vi "Main.vi"() -> ()   [LabVIEW 2018] (continued)
                n2266 = Insert Into Array(array=string[] [] ("数组"), index=0 ("索引"), new element #1=w3062, new element #2=w3061, new element #3=w3060) -> (w3066:string[])
                n2267 = Bundle By Name(cluster=cluster{"Data":string[], "State":T1} {"Data"=[], "State"=enum."PLC通讯初始化"} ("元素"), "Data"=w3066, "State"=状态2."扫码回复") -> (w3067:cluster{"Data":string[], "State":T1})
                n2268 = Enqueue Element(queue=w3056, element=w3067) -> ()  [unwired: 2 in, 3 out]
              }
            }
            n2269 = Unbundle By Name(w2986) -> ("source"=w2985:string)
            n2270 = Concatenate Strings("80扫码异常 ", w2985) -> (w2983:string)
            "ST80扫码请求(事件)" <- FALSE ("ST80扫码请求(事件)")
          }
          event "查询": Value Change {
            n2271 = event-data() -> ()  [unwired: 1 in, 2 out]
            n2272 = flat-sequence {
              tunnel: w3083 -> [w3108]
              tunnel: w3082 -> [w3107]
              tunnel: [w3099] -> w3081
              frame #0 {
                w3084 = cluster{u32, u32}[] [{1985280, 1985280}, {6618880, 6618880}, {1985280, 1985280}, {6618880, 6618880}] ("颜色[4]")
                n2273 = property on="101" class="Bool (严格)"("Colors [4]"=w3084) -> ()  [unwired: 2 in, 2 out]
                n2274 = property on="102" class="Bool (严格)"("Colors [4]"=w3084) -> ()  [unwired: 2 in, 2 out]
                n2275 = property on="202" class="Bool (严格)"("Colors [4]"=w3084) -> ()  [unwired: 2 in, 2 out]
                n2276 = property on="203" class="Bool (严格)"("Colors [4]"=w3084) -> ()  [unwired: 2 in, 2 out]
                n2277 = property on="301" class="Bool (严格)"("Colors [4]"=w3084) -> ()  [unwired: 2 in, 2 out]
                n2278 = property on="302" class="Bool (严格)"("Colors [4]"=w3084) -> ()  [unwired: 2 in, 2 out]
                n2279 = property on="401" class="Bool (严格)"("Colors [4]"=w3084) -> ()  [unwired: 2 in, 2 out]
                n2280 = property on="403" class="Bool (严格)"("Colors [4]"=w3084) -> ()  [unwired: 2 in, 2 out]
                n2281 = property on="502" class="Bool (严格)"("Colors [4]"=w3084) -> ()  [unwired: 2 in, 2 out]
                n2282 = property on="503" class="Bool (严格)"("Colors [4]"=w3084) -> ()  [unwired: 2 in, 2 out]
                n2283 = property on="601" class="Bool (严格)"("Colors [4]"=w3084) -> ()  [unwired: 2 in, 2 out]
                n2284 = property on="602" class="Bool (严格)"("Colors [4]"=w3084) -> ()  [unwired: 2 in, 2 out]
                n2285 = property on="70" class="Bool (严格)"("Colors [4]"=w3084) -> ()  [unwired: 2 in, 2 out]
                n2286 = property on="80" class="Bool (严格)"("Colors [4]"=w3084) -> ()  [unwired: 2 in, 2 out]
              }
              frame #1 {
                n2287 = Concatenate Strings("Where QRCode='" ("查询语句"), "输入需要Rework的一维码：", "'" ("字符串")) -> (w3109:string)
                n2288 = call "SQL_Select.vi"("要读取的列名"=string[] ["Last_Station", "Last_Result"] ("列名"), "表名"="Online", "error in (no error)"=w3107, "查询语句"=w3109, "查询条件"=TRUE, "connection reference"=w3108) -> ("error out"=w3099:errorcluster, "数据"=w3104:string[][])  [unwired: 3 in, 1 out]
                n2289 = Index Array(array=w3104, index (row)=0 ("索引 (行)")) -> (element=w3102:string[])  [unwired: 1 in]
                n2290 = Index Array(array=w3102) -> (element #1=w3101:string, element #2=w3100:string)  [unwired: 2 in]
                n2291 = case shown="\"0\", 默认" w3101 {
                  tunnel: w3100 -> [_ w3117 w3124 w3131 w3138 w3145 w3152 w3159 w3166 w3173 w3180 w3187 w3194 w3201 w3207]
                  tunnel: [w3114 w3116 TRUE w3129 w3136 w3143 w3150 w3157 w3164 w3171 w3178 w3185 w3192 w3199 w3205] -> w3098
                  tunnel: [w3114 w3115 w3123 w3129 w3136 w3143 w3150 w3157 w3164 w3171 w3178 w3185 w3192 w3199 w3205] -> w3097
                  tunnel: [w3114 w3115 w3121 w3130 w3136 w3143 w3150 w3157 w3164 w3171 w3178 w3185 w3192 w3199 w3205] -> w3096
                  tunnel: [w3114 w3115 w3121 w3128 w3137 w3143 w3150 w3157 w3164 w3171 w3178 w3185 w3192 w3199 w3205] -> w3095
                  tunnel: [w3114 w3115 w3121 w3128 w3135 w3144 w3150 w3157 w3164 w3171 w3178 w3185 w3192 w3199 w3205] -> w3094
                  tunnel: [w3114 w3115 w3121 w3128 w3135 w3142 w3151 w3157 w3164 w3171 w3178 w3185 w3192 w3199 w3205] -> w3093
                  tunnel: [w3114 w3115 w3121 w3128 w3135 w3142 w3149 w3158 w3164 w3171 w3178 w3185 w3192 w3199 w3205] -> w3092
                  tunnel: [w3114 w3115 w3121 w3128 w3135 w3142 w3149 w3156 w3165 w3171 w3178 w3185 w3192 w3199 w3205] -> w3091
                  tunnel: [w3114 w3115 w3121 w3128 w3135 w3142 w3149 w3156 w3163 w3172 w3178 w3185 w3192 w3199 w3205] -> w3090
                  tunnel: [w3114 w3115 w3121 w3128 w3135 w3142 w3149 w3156 w3163 w3170 w3179 w3185 w3192 w3199 w3205] -> w3089
                  tunnel: [w3114 w3115 w3121 w3128 w3135 w3142 w3149 w3156 w3163 w3170 w3177 w3186 w3192 w3199 w3205] -> w3088
                  tunnel: [w3114 w3115 w3121 w3128 w3135 w3142 w3149 w3156 w3163 w3170 w3177 w3184 w3193 w3199 w3205] -> w3087
                  tunnel: [w3114 w3115 w3121 w3128 w3135 w3142 w3149 w3156 w3163 w3170 w3177 w3184 w3191 w3200 w3205] -> w3086
                  tunnel: [w3114 w3115 w3121 w3128 w3135 w3142 w3149 w3156 w3163 w3170 w3177 w3184 w3191 FALSE w3206] -> w3085
                  frame "0", Default {
                    w3114 = FALSE
                  }
                  frame "101" {
                    w3115 = FALSE
                    n2292 = case shown="\"OK\", 默认" w3117 {
                      tunnel: [TRUE FALSE] -> w3116
                      frame "OK", Default {
                      }
                      frame "NG" {
                        n2293 = property on="101" class="Bool (严格)"("Colors [4]"=cluster{u32, u32}[] [{16711680, 16711680}, {6618880, 6618880}, {1985280, 1985280}, {6618880, 6618880}] ("颜色[4]")) -> ()  [unwired: 2 in, 2 out]
                      }
                    }
                  }
                  frame "102" {
                    w3121 = FALSE
                    n2294 = case shown="\"NG\"" w3124 {
                      tunnel: [TRUE FALSE] -> w3123
                      frame "OK", Default {
                      }
                      frame "NG" {
                        n2295 = property on="102" class="Bool (严格)"("Colors [4]"=cluster{u32, u32}[] [{16711680, 16711680}, {6618880, 6618880}, {1985280, 1985280}, {6618880, 6618880}] ("颜色[4]")) -> ()  [unwired: 2 in, 2 out]
                      }
                    }
                  }
                  frame "202" {
                    w3129 = TRUE
                    w3128 = FALSE
                    n2296 = case shown="\"NG\"" w3131 {
                      tunnel: [TRUE FALSE] -> w3130
                      frame "OK", Default {
                      }
                      frame "NG" {
                        n2297 = property on="202" class="Bool (严格)"("Colors [4]"=cluster{u32, u32}[] [{16711680, 16711680}, {6618880, 6618880}, {1985280, 1985280}, {6618880, 6618880}] ("颜色[4]")) -> ()  [unwired: 2 in, 2 out]
                      }
                    }
                  }
                  frame "203" {
                    w3136 = TRUE
                    w3135 = FALSE
                    n2298 = case shown="\"NG\"" w3138 {
                      tunnel: [TRUE FALSE] -> w3137
                      frame "OK", Default {
                      }
                      frame "NG" {
                        n2299 = property on="203" class="Bool (严格)"("Colors [4]"=cluster{u32, u32}[] [{16711680, 16711680}, {6618880, 6618880}, {1985280, 1985280}, {6618880, 6618880}] ("颜色[4]")) -> ()  [unwired: 2 in, 2 out]
                      }
                    }
                  }
                  frame "301" {
                    w3143 = TRUE
                    w3142 = FALSE
                    n2300 = case shown="\"NG\"" w3145 {
                      tunnel: [TRUE FALSE] -> w3144
                      frame "OK", Default {
                      }
                      frame "NG" {
                        n2301 = property on="301" class="Bool (严格)"("Colors [4]"=cluster{u32, u32}[] [{16711680, 16711680}, {6618880, 6618880}, {1985280, 1985280}, {6618880, 6618880}] ("颜色[4]")) -> ()  [unwired: 2 in, 2 out]
                      }
                    }
                  }
                  frame "302" {
                    w3150 = TRUE
                    w3149 = FALSE
                    n2302 = case shown="\"NG\"" w3152 {
                      tunnel: [TRUE FALSE] -> w3151
                      frame "OK", Default {
                      }
                      frame "NG" {
                        n2303 = property on="302" class="Bool (严格)"("Colors [4]"=cluster{u32, u32}[] [{16711680, 16711680}, {6618880, 6618880}, {1985280, 1985280}, {6618880, 6618880}] ("颜色[4]")) -> ()  [unwired: 2 in, 2 out]
                      }
                    }
                  }
                  frame "401" {
                    w3157 = TRUE
                    w3156 = FALSE
                    n2304 = case shown="\"NG\"" w3159 {
                      tunnel: [TRUE FALSE] -> w3158
                      frame "OK", Default {
                      }
                      frame "NG" {
                        n2305 = property on="401" class="Bool (严格)"("Colors [4]"=cluster{u32, u32}[] [{16711680, 16711680}, {6618880, 6618880}, {1985280, 1985280}, {6618880, 6618880}] ("颜色[4]")) -> ()  [unwired: 2 in, 2 out]
                      }
                    }
                  }
                  frame "403" {
                    w3163 = FALSE
                    w3164 = TRUE
                    n2306 = case shown="\"NG\"" w3166 {
                      tunnel: [TRUE FALSE] -> w3165
                      frame "OK", Default {
                      }
                      frame "NG" {
                        n2307 = property on="403" class="Bool (严格)"("Colors [4]"=cluster{u32, u32}[] [{16711680, 16711680}, {6618880, 6618880}, {1985280, 1985280}, {6618880, 6618880}] ("颜色[4]")) -> ()  [unwired: 2 in, 2 out]
                      }
                    }
                  }
                  frame "502" {
                    w3170 = FALSE
                    w3171 = TRUE
                    n2308 = case shown="\"NG\"" w3173 {
                      tunnel: [TRUE FALSE] -> w3172
                      frame "OK", Default {
                      }
                      frame "NG" {
                        n2309 = property on="502" class="Bool (严格)"("Colors [4]"=cluster{u32, u32}[] [{16711680, 16711680}, {6618880, 6618880}, {1985280, 1985280}, {6618880, 6618880}] ("颜色[4]")) -> ()  [unwired: 2 in, 2 out]
                      }
                    }
                  }
                  frame "503" {
                    w3177 = FALSE
                    w3178 = TRUE
                    n2310 = case shown="\"NG\"" w3180 {
                      tunnel: [TRUE FALSE] -> w3179
                      frame "OK", Default {
                      }
                      frame "NG" {
                        n2311 = property on="503" class="Bool (严格)"("Colors [4]"=cluster{u32, u32}[] [{16711680, 16711680}, {6618880, 6618880}, {1985280, 1985280}, {6618880, 6618880}] ("颜色[4]")) -> ()  [unwired: 2 in, 2 out]
                      }
                    }
                  }
                  frame "601" {
                    w3184 = FALSE
                    w3185 = TRUE
                    n2312 = case shown="\"NG\"" w3187 {
                      tunnel: [TRUE FALSE] -> w3186
                      frame "OK", Default {
                      }
                      frame "NG" {
                        n2313 = property on="601" class="Bool (严格)"("Colors [4]"=cluster{u32, u32}[] [{16711680, 16711680}, {6618880, 6618880}, {1985280, 1985280}, {6618880, 6618880}] ("颜色[4]")) -> ()  [unwired: 2 in, 2 out]
                      }
                    }
                  }
                  frame "602" {
                    w3191 = FALSE
                    w3192 = TRUE
                    n2314 = case shown="\"NG\"" w3194 {
                      tunnel: [TRUE FALSE] -> w3193
                      frame "OK", Default {
                      }
                      frame "NG" {
                        n2315 = property on="602" class="Bool (严格)"("Colors [4]"=cluster{u32, u32}[] [{16711680, 16711680}, {6618880, 6618880}, {1985280, 1985280}, {6618880, 6618880}] ("颜色[4]")) -> ()  [unwired: 2 in, 2 out]
                      }
                    }
                  }
                  frame "70" {
                    w3199 = TRUE
                    n2316 = case shown="\"NG\"" w3201 {
                      tunnel: [TRUE FALSE] -> w3200
                      frame "OK", Default {
                      }
                      frame "NG" {
                        n2317 = property on="70" class="Bool (严格)"("Colors [4]"=cluster{u32, u32}[] [{16711680, 16711680}, {6618880, 6618880}, {1985280, 1985280}, {6618880, 6618880}] ("颜色[4]")) -> ()  [unwired: 2 in, 2 out]
                      }
                    }
                  }
                  frame "80" {
                    w3205 = TRUE
                    n2318 = case shown="\"NG\"" w3207 {
                      tunnel: [TRUE FALSE] -> w3206
                      frame "OK", Default {
                      }
                      frame "NG" {
                        n2319 = property on="80" class="Bool (严格)"("Colors [4]"=cluster{u32, u32}[] [{16711680, 16711680}, {6618880, 6618880}, {1985280, 1985280}, {6618880, 6618880}] ("颜色[4]")) -> ()  [unwired: 2 in, 2 out]
                      }
                    }
                  }
                }
                n2320 = local write "101"(w3098) -> ()
                n2321 = local write "102"(w3097) -> ()
                n2322 = local write "202"(w3096) -> ()
                n2323 = local write "203"(w3095) -> ()
                n2324 = local write "301"(w3094) -> ()
                n2325 = local write "302"(w3093) -> ()
                n2326 = local write "401"(w3092) -> ()
                n2327 = local write "403"(w3091) -> ()
                n2328 = local write "502"(w3090) -> ()
                n2329 = local write "503"(w3089) -> ()
                n2330 = local write "601"(w3088) -> ()
                n2331 = local write "602"(w3087) -> ()
                n2332 = local write "70"(w3086) -> ()
                n2333 = local write "80"(w3085) -> ()
              }
            }
          }
          event "确定Rework": Value Change {
            n2334 = event-data() -> ()  [unwired: 1 in, 2 out]
            n2335 = stacked-sequence {
              seq-local: [w3215 _] -> [_ w3241]
              tunnel: w3214 -> [w3225 w3246]
              tunnel: w3213 -> [w3224 w3245]
              tunnel: [_ w3244] -> w3212
              frame #0 {
                n2336 = local read "输入需要Rework的一维码："() -> (w3220:string)
                n2337 = Concatenate Strings("Where QRCode='" ("查询语句"), w3220, "'" ("字符串")) -> (w3219:string)
                n2338 = call "SQL_Select.vi"("表名"="Online", "error in (no error)"=w3224, "查询语句"=w3219, "查询条件"=TRUE, "connection reference"=w3225) -> ("数据"=w3218:string[][])  [unwired: 4 in, 2 out]
                n2339 = Matrix Size(0:w3218) -> (1:w3217:i32)  [unwired: 1 out]
                n2340 = Equal?(x=w3217, y=0) -> (x = y?=w3215:bool)
              }
              frame #1 {
                n2341 = Insert Into Array(array=bool[] [] ("数组"), index=0 ("索引"), new element #1="70", new element #2="602", new element #3="601", new element #4="503", new element #5="502", new element #6="403", new element #7="401", new element #8="302", new element #9="301", new element #10="203", new element #11="202", new element #12="102", new element #13="101", new element #14="80") -> (w3250:bool[])
                n2342 = Search 1D Array(1D array=w3250, element=TRUE ("元素")) -> (index of element=w3247:i32)  [unwired: 1 in]
                n2343 = Equal?(x=w3247, y=-1) -> (x = y?=w3243:bool)
                n2344 = Or(x=w3243, y=w3241) -> (x .or. y?=w3242:bool)
                n2345 = case shown="假" w3242 {
                  tunnel: w3247 -> [w3290 _]
                  tunnel: w3246 -> [w3289 _]
                  tunnel: w3245 -> [w3288 w3392]
                  tunnel: [w3258 w3392] -> w3244
                  frame False {
                    w3263 = "Rework_List" ("表名")
                    w3261 = 0 ("索引 (行)")
                    w3273 = "Online" ("表名")
                    n2346 = case shown="13" w3290 {
                      tunnel: w3289 -> [w3351 w3353 w3357 w3360 w3363 w3366 w3369 w3372 w3375 w3378 w3381 w3384 w3386 w3389]
                      tunnel: w3288 -> [w3350 w3352 w3356 w3359 w3362 w3365 w3368 w3371 w3374 w3377 w3380 w3383 w3385 w3388]
                      tunnel: [w3350 w3352 w3356 w3359 w3362 w3365 w3368 w3371 w3374 w3377 w3380 w3383 w3385 w3388] -> w3276
                      tunnel: [w3351 w3353 w3357 w3360 w3363 w3366 w3369 w3372 w3375 w3378 w3381 w3384 w3386 w3389] -> w3277
                      tunnel: ["70" "602" "601" "503" "502" "403" "401" "302" "301" "203" "202" "102" "101" "80"] -> w3253
                      frame 0, Default {
                      }
                      frame 1 {
                      }
                      frame 2 {
                      }
                      frame 3 {
                      }
                      frame 4 {
                      }
                      frame 5 {
                      }
                      frame 6 {
                      }
                      frame 7 {
                      }
                      frame 8 {
                      }
                      frame 9 {
                      }
                      frame 10 {
                      }
                      frame 11 {
                      }
                      frame 12 {
                      }
                      frame 13 {
                      }
                    }
                    n2347 = local read "输入需要Rework的一维码："() -> (w3259:string)
                    n2348 = Concatenate Strings("Where QRCode='" ("查询语句"), w3259, "'" ("字符串")) -> (w3260:string)
                    n2349 = call "SQL_Select.vi"("要读取的列名"=string[] ["Last_Station"], "表名"=w3273, "error in (no error)"=w3276, "查询语句"=w3260, "查询条件"=TRUE, "connection reference"=w3277) -> ("error out"=w3274:errorcluster, "数据"=w3272:string[][], "connection reference out"=w3275:T12)  [unwired: 3 in]
                    n2350 = Index Array(array=w3272, index (row)=w3261, index (col)=w3261) -> (element=w3254:string)
                    n2351 = Insert Into Array(array=string[] [] ("数组"), index=0 ("索引"), new element #1=w3253, new element #2="OK" ("新元素/子数组"), new element #3="T" ("新元素/子数组")) -> (w3286:string[])
                    n2352 = call "SQL_Update.vi"("查询语句"=w3260, "表名"=w3273, "error in (no error)"=w3274, "列名对应的值"=w3286, "列名"=string[] ["Last_Station", "Last_Result", "Rework_Status"], "connection reference"=w3275) -> ("error out"=w3271:errorcluster, "connection reference 2"=w3270:T12)  [unwired: 4 in]
                    n2353 = call "SQL_Select.vi"("表名"=w3263, "error in (no error)"=w3271, "查询语句"=w3260, "查询条件"=TRUE, "connection reference"=w3270) -> ("error out"=w3264:errorcluster, "数据"=w3268:string[][], "connection reference out"=w3265:T12)  [unwired: 4 in]
                    n2354 = call "Rework_Calculate-1.vi"("Rework站号"=w3253, "当前站号"=w3254) -> ("Data"=w3255:string[], "Rework_List"=w3256:string[], "跨站"=w3257:bool)  [unwired: 7 in]
                    n2355 = Matrix Size(0:w3268) -> (1:w3267:i32)  [unwired: 1 out]
                    n2356 = Equal To 0?(x=w3267) -> (x = 0?=w3266:bool)
                    n2357 = case shown="假" w3257 {
                      tunnel: w3266 -> [w3309 _]
                      tunnel: w3265 -> [w3308 w3345]
                      tunnel: w3264 -> [w3307 w3346]
                      tunnel: w3255 -> [w3306 _]
                      tunnel: w3256 -> [w3305 _]
                      tunnel: w3263 -> [w3304 _]
                      tunnel: w3260 -> [w3300 _]
                      tunnel: w3259 -> [w3293 _]
                      tunnel: [w3292 w3346] -> w3258
                      tunnel: [w3291 w3345] -> _
                      frame False {
                        w3294 = "Rework" ("表名")
                        n2358 = case shown="真" w3309 {
                          tunnel: w3308 -> [w3331 w3344]
                          tunnel: w3307 -> [w3330 w3343]
                          tunnel: w3306 -> [w3328 w3338]
                          tunnel: w3305 -> [w3329 w3341]
                          tunnel: w3304 -> [w3327 w3342]
                          tunnel: w3293 -> [_ w3336]
                          tunnel: [w3325 w3333] -> w3302
                          tunnel: [w3324 w3332] -> w3301
                          tunnel: w3300 -> [w3326 _]
                          frame False {
                            n2359 = call "SQL_Update.vi"("查询语句"=w3326, "表名"=w3327, "error in (no error)"=w3330, "列名对应的值"=w3328, "列名"=w3329, "connection reference"=w3331) -> ("error out"=w3324:errorcluster, "connection reference 2"=w3325:T12)  [unwired: 4 in]
                          }
                          frame True {
                            n2360 = Insert Into Array(array=w3341, index=0 ("索引"), new element="QRCode" ("新元素/子数组")) -> (w3335:string[])
                            n2361 = Insert Into Array(array=w3338, index=0 ("索引"), new element=w3336) -> (w3334:string[])
                            n2362 = call "SQL_Insert.vi"("表名"=w3342, "error in (no error)"=w3343, "值"=w3334, "列名"=w3335, "connection reference"=w3344) -> ("error out"=w3332:errorcluster, "connection reference 2"=w3333:T12)  [unwired: 5 in]
                          }
                        }
                        n2363 = call "SQL_Select.vi"("表名"=w3294, "error in (no error)"=w3301, "查询语句"=w3300, "查询条件"=TRUE, "connection reference"=w3302) -> ("error out"=w3295:errorcluster, "数据"=w3299:string[][], "connection reference out"=w3296:T12)  [unwired: 4 in]
                        n2364 = Matrix Size(0:w3299) -> (1:w3298:i32)  [unwired: 1 out]
                        n2365 = Equal To 0?(x=w3298) -> (x = 0?=w3297:bool)
                        n2366 = case shown="真" w3297 {
                          tunnel: w3296 -> [w3310 w3323]
                          tunnel: w3295 -> [w3311 w3322]
                          tunnel: w3294 -> [_ w3321]
                          tunnel: w3293 -> [_ w3319]
                          tunnel: [w3311 w3315] -> w3292
                          tunnel: [w3310 w3312] -> w3291
                          frame False {
                          }
                          frame True {
                            n2367 = Format Date/Time String(time format string (%c)="%Y-%m-%d_%H:%M" ("时间格式字符串(%c)")) -> (date/time string=w3313:string)  [unwired: 2 in]
                            n2368 = Insert Into Array(array=string[] [] ("数组"), index=0 ("索引"), new element #1=w3319, new element #2=w3313) -> (w3316:string[])
                            n2369 = call "SQL_Insert.vi"("表名"=w3321, "error in (no error)"=w3322, "值"=w3316, "列名"=string[] ["QRCode", "Online_Time"], "connection reference"=w3323) -> ("error out"=w3315:errorcluster, "connection reference 2"=w3312:T12)  [unwired: 5 in]
                          }
                        }
                      }
                      frame True {
                      }
                    }
                    n2370 = case shown="错误" w3258 {
                      tunnel: ["Rework成功！" ("Rework状态") "Rework失败！" ("Rework状态")] -> w3262
                      frame No Error {
                      }
                      frame Error {
                      }
                    }
                    "Rework状态" <- w3262
                  }
                  frame True {
                    n2371 = local write "Rework状态"("该条码不存在！" ("Rework状态")) -> ()
                  }
                }
              }
            }
          }
        }
        n2372 = event shown="[2] \"ST70数据读取(事件)\": 值改变" {
          selector: _ -> [_ _ _]
          dyn-events: _ -> [_ _ _]
          timeout: 10 -> [_ _ _]
          tunnel: w763 -> [_ w788 w836]
          tunnel: w762 -> [_ w787 w835]
          tunnel: w761 -> [_ w786 w837]
          tunnel: w760 -> [_ _ w838]
          event Timeout {
            n2373 = event-data() -> ()  [unwired: 1 in, 3 out]
          }
          event "ST70扫码请求(事件)": Value Change {
            n2374 = event-data() -> ()  [unwired: 1 in, 1 out]
            n2375 = local read "70二维码"() -> (w815:string)
            n2376 = Concatenate Strings("Where QRCode='" ("查询语句"), w815, "'" ("字符串")) -> (w803:string)
            n2377 = call "SQL_Select.vi"("要读取的列名"=string[] ["Last_Station", "Last_Result"], "表名"="Online", "error in (no error)"=w787, "查询语句"=w803, "查询条件"=TRUE, "connection reference"=w788) -> ("error out"=w784:errorcluster, "数据"=w804:string[][])  [unwired: 3 in, 1 out]
            n2378 = case shown="无错误" w784 {
              tunnel: w804 -> [w831 _]
              tunnel: ["1" ("右扫码请求回复") "2" ("右扫码请求回复")] -> w807
              tunnel: [w826 w832] -> w808
              tunnel: [w825 w832] -> w809
              frame No Error {
                n2379 = Index Array(array=w831, index (row)=0 ("索引 (行)")) -> (element=w828:string[])  [unwired: 1 in]
                n2380 = Index Array(array=w828, index #1=0 ("索引 (行)")) -> (element #1=w826:string, element #2=w825:string)  [unwired: 1 in]
                "上一站号 (70)" <- w826
                "上一站结果 (70)" <- w825
              }
              frame Error {
                w832 = ""
              }
            }
            n2381 = Insert Into Array(array=string[] [] ("数组"), index=0 ("索引"), new element #1=w807, new element #2=w808, new element #3=w809) -> (w806:string[])
            n2382 = Format Date/Time String(time format string (%c)="%Y-%m-%d" ("时间格式字符串(%c)")) -> (date/time string=w810:string)  [unwired: 2 in]
            n2383 = Get Date/Time String() -> (time string=w811:string)  [unwired: 3 in, 1 out]
            n2384 = Bundle By Name(cluster=cluster{"Data":string[], "State":T1} {"Data"=[], "State"=enum."PLC通讯初始化"} ("元素"), "Data"=w806, "State"=状态2."扫码回复") -> (w805:cluster{"Data":string[], "State":T1})
            n2385 = Insert Into Array(array=string[] [] ("数组"), index=0 ("索引"), new element #1=w810, new element #2=w811, new element #3=w815) -> (w812:string[])
            n2386 = Enqueue Element(queue=w786, element=w805) -> ()  [unwired: 2 in, 3 out]
            n2387 = Insert Into Array(array=string[][] [] ("数组"), index (row)=0 ("索引 (行)"), new element=w812) -> (w813:string[][])  [unwired: 1 in]
            n2388 = Transpose 2D Array(2D array=w813) -> (transposed array=w814:string[][])
            n2389 = property on="ST70_DATA" class="MCListbox (严格)"("ItemNames"=w814) -> ()  [unwired: 2 in, 2 out]
            n2390 = case shown="错误" w784 {
              tunnel: "ST70 扫码请求错误" -> [_ w821]
              frame No Error {
              }
              frame Error {
                n2391 = property on="错误信息" class="LstBox (严格)"() -> ("Item Names"=w820:string[])  [unwired: 2 in, 2 out]
                n2392 = Format Date/Time String(time format string (%c)="%Y-%m-%d %H:%M:%S" ("时间格式字符串(%c)")) -> (date/time string=w823:string)  [unwired: 2 in]
                n2393 = Concatenate Strings(w823, "  " ("字符串"), w821) -> (w818:string)
                n2394 = Insert Into Array(array=w820, index=0 ("索引"), new element=w818) -> (w817:string[])
                n2395 = property on="错误信息" class="LstBox (严格)"("Item Names"=w817) -> ()  [unwired: 2 in, 2 out]
              }
            }
            "ST70扫码请求(事件)" <- FALSE ("ST70扫码请求(事件)")
          }
          event "ST70数据读取(事件)": Value Change {
            w854 = 0 ("索引 (行)")
            # "数据库操作"
            n2396 = event-data() -> ()  [unwired: 1 in, 1 out]
            n2397 = Dequeue Element(queue=w838, timeout in ms (-1)=10 ("超时毫秒(-1)")) -> (element=w867:string[])  [unwired: 1 in, 3 out]
            n2398 = local read "70二维码"() -> (w870:string)
            n2399 = Concatenate Strings("Where QRCode='" ("查询语句"), w870, "'" ("字符串")) -> (w869:string)
            n2400 = call "SQL_Select.vi"("要读取的列名"=string[] ["Rework_Status"], "表名"="Online", "error in (no error)"=w835, "查询语句"=w869, "查询条件"=TRUE, "connection reference"=w836) -> ("error out"=w865:errorcluster, "数据"=w861:string[][], "connection reference out"=w864:T12)  [unwired: 3 in]
            n2401 = Index Array(array=w861, index (row)=w854, index (col)=w854) -> (element=w862:string)
            n2402 = Equal?(x=w862, y="T") -> (x = y?=w863:bool)
            n2403 = case shown="真" w863 {
              tunnel: [w884 w889] -> w866
              tunnel: w867 -> [w883 w892]
              tunnel: [w878 w888] -> w834
              tunnel: w870 -> [w877 w891]
              tunnel: w869 -> [w873 w890]
              tunnel: w864 -> [w876 w903]
              tunnel: w865 -> [w875 w902]
              frame False {
                n2404 = call "SQL_Update.vi"("查询语句"=w873, "表名"="Online", "error in (no error)"=w875, "列名对应的值"=w883, "列名"=string[] ["Last_Station", "Last_Result", "ST70_Date", "ST70_Time", "ST70_Package_Result", "Marking_Code", "ST70_Marking_Code_Class", "ST70_Force", "ST70_Force_Upper", "ST70_Force_Lower", "ST70_Displacement", "ST70_Displacement_Upper", "ST70_Displacement_Lower", "ST70_Shaft_Seal_5024366", "ST70_Camera_Shield", "ST70_Process_Pressure_Max", "ST70_Process_Pressure_Upper", "ST70_Process_Pressure_Lower"], "connection reference"=w876) -> ("error out"=w878:errorcluster)  [unwired: 4 in, 1 out]
                n2405 = Unbundle By Name(w878) -> ("status"=w882:bool)
                n2406 = Equal?(x=w877, y="") -> (x = y?=w880:bool)
                n2407 = Or(x=w882, y=w880) -> (x .or. y?=w879:bool)
                n2408 = case shown="假" w879 {
                  tunnel: ["1" ("数据保存请求回复") "2" ("数据保存请求回复")] -> w884
                  frame False {
                  }
                  frame True {
                  }
                }
              }
              frame True {
                w898 = 0 ("索引 (行)")
                n2409 = call "SQL_Select.vi"("要读取的列名"=string[] ["[70]"], "表名"="Rework_List", "error in (no error)"=w902, "查询语句"=w890, "查询条件"=TRUE, "connection reference"=w903) -> ("error out"=w893:errorcluster, "数据"=w899:string[][], "connection reference out"=w894:T12)  [unwired: 3 in]
                n2410 = Index Array(array=w899, index (row)=w898, index (col)=w898) -> (element=w897:string)
                n2411 = Equal?(x=w897, y="T") -> (x = y?=w895:bool)
                n2412 = case shown="真" w895 {
                  tunnel: w894 -> [w911 w930]
                  tunnel: w893 -> [w912 w929]
                  tunnel: w892 -> [w910 w936]
                  tunnel: w891 -> [w907 w931]
                  tunnel: w890 -> [w909 w921]
                  tunnel: [w906 w923] -> w889
                  tunnel: [w908 w922] -> w888
                  frame False {
                    n2413 = call "SQL_Update.vi"("查询语句"=w909, "表名"="Online", "error in (no error)"=w912, "列名对应的值"=w910, "列名"=string[] ["Last_Station", "Last_Result", "ST70_Date", "ST70_Time", "ST70_Package_Result", "Marking_Code", "ST70_Marking_Code_Class", "ST70_Force", "ST70_Force_Upper", "ST70_Force_Lower", "ST70_Displacement", "ST70_Displacement_Upper", "ST70_Displacement_Lower", "ST70_Shaft_Seal_5024366", "ST70_Camera_Shield", "ST70_Process_Pressure_Max", "ST70_Process_Pressure_Upper", "ST70_Process_Pressure_Lower"], "connection reference"=w911) -> ("error out"=w908:errorcluster)  [unwired: 4 in, 1 out]
                    n2414 = Unbundle By Name(w908) -> ("status"=w916:bool)
                    n2415 = Equal?(x=w907, y="") -> (x = y?=w914:bool)
                    n2416 = Or(x=w916, y=w914) -> (x .or. y?=w913:bool)
                    n2417 = case shown="假" w913 {
                      tunnel: ["1" ("数据保存请求回复") "2" ("数据保存请求回复")] -> w906
                      frame False {
                      }
                      frame True {
                      }
                    }
                  }
                  frame True {
                    n2418 = Delete From Array(array=w936, length=2 ("长度"), index=0 ("索引")) -> (deleted portion=w924:string[], array with subset deleted=w933:string[])
                    n2419 = call "SQL_Update.vi"("查询语句"=w921, "表名"="Online", "error in (no error)"=w929, "列名对应的值"=w924, "列名"=string[] ["Last_Station", "Last_Result"], "connection reference"=w930) -> ("error out"=w928:errorcluster, "connection reference 2"=w927:T12)  [unwired: 4 in]
                    n2420 = call "SQL_Update.vi"("查询语句"=w921, "表名"="Rework", "error in (no error)"=w928, "列名对应的值"=w933, "列名"=string[] ["ST70_Date", "ST70_Time", "ST70_Package_Result", "Marking_Code", "ST70_Marking_Code_Class", "ST70_Force", "ST70_Force_Upper", "ST70_Force_Lower", "ST70_Displacement", "ST70_Displacement_Upper", "ST70_Displacement_Lower", "ST70_Shaft_Seal_5024366", "ST70_Camera_Shield", "ST70_Process_Pressure_Max", "ST70_Process_Pressure_Upper", "ST70_Process_Pressure_Lower"], "connection reference"=w927) -> ("error out"=w922:errorcluster)  [unwired: 4 in, 1 out]
                    n2421 = Unbundle By Name(w922) -> ("status"=w939:bool)
                    n2422 = Equal?(x="", y=w931) -> (x = y?=w938:bool)
                    n2423 = Or(x=w939, y=w938) -> (x .or. y?=w937:bool)
                    n2424 = case shown="真" w937 {
                      tunnel: ["1" ("数据保存请求回复") "2" ("数据保存请求回复")] -> w923
                      frame False {
                      }
                      frame True {
                      }
                    }
                  }
                }
              }
            }
            n2425 = Insert Into Array(array=string[] [] ("数组"), index=0 ("索引"), new element=w866) -> (w856:string[])
            n2426 = Bundle By Name(cluster=cluster{"Data":string[], "State":T1} {"Data"=[], "State"=enum."PLC通讯初始化"} ("元素"), "Data"=w856, "State"=状态2."数据保存回复") -> (w857:cluster{"Data":string[], "State":T1})
            n2427 = Delete From Array(array=w867, length=2 ("长度"), index=0 ("索引")) -> (array with subset deleted=w859:string[])  [unwired: 1 out]
            n2428 = Enqueue Element(queue=w837, element=w857) -> ()  [unwired: 2 in, 3 out]
            n2429 = Insert Into Array(array=w859, index=2 ("索引"), new element=w870) -> (w860:string[])
            n2430 = Insert Into Array(array=string[][] [] ("数组"), index (row)=0 ("索引 (行)"), new element=w860) -> (w858:string[][])  [unwired: 1 in]
            n2431 = Transpose 2D Array(2D array=w858) -> (transposed array=w868:string[][])
            n2432 = property on="ST70_DATA" class="MCListbox (严格)"("ItemNames"=w868) -> ()  [unwired: 2 in, 2 out]
            n2433 = case shown="错误" w834 {
              tunnel: "ST70 数据读取错误" -> [_ w947]
              frame No Error {
              }
              frame Error {
                n2434 = property on="错误信息" class="LstBox (严格)"() -> ("Item Names"=w946:string[])  [unwired: 2 in, 2 out]
                n2435 = Format Date/Time String(time format string (%c)="%Y-%m-%d %H:%M:%S" ("时间格式字符串(%c)")) -> (date/time string=w949:string)  [unwired: 2 in]
                n2436 = Concatenate Strings(w949, "  " ("字符串"), w947) -> (w944:string)
                n2437 = Insert Into Array(array=w946, index=0 ("索引"), new element=w944) -> (w943:string[])
                n2438 = property on="错误信息" class="LstBox (严格)"("Item Names"=w943) -> ()  [unwired: 2 in, 2 out]
              }
            }
            "ST70数据读取(事件)" <- FALSE ("ST70数据读取(事件)")
          }
        }
        n2439 = local read "退出"() -> (w781:bool)
        n2440 = case shown="错误" w767 {
          selector: w767 -> [_ w952]
          tunnel: w768 -> [_ w958]
          frame No Error {
          }
          frame Error {
            w953 = "  " ("字符串")
            n2441 = property on="错误信息" class="LstBox (严格)"() -> ("Item Names"=w957:string[])  [unwired: 2 in, 2 out]
            n2442 = Unbundle By Name(w952) -> ("source"=w951:string)
            n2443 = Format Date/Time String(time format string (%c)="%Y-%m-%d %H:%M:%S" ("时间格式字符串(%c)")) -> (date/time string=w959:string)  [unwired: 2 in]
            n2444 = Concatenate Strings(w959, w953, w958, w953, w951) -> (w955:string)
            n2445 = Insert Into Array(array=w957, index=0 ("索引"), new element=w955) -> (w954:string[])
            n2446 = property on="错误信息" class="LstBox (严格)"("Item Names"=w954) -> ()  [unwired: 2 in, 2 out]
          }
        }
        n2447 = Wait (ms)(milliseconds to wait=u32 10 ("等待时间（毫秒）")) -> ()  [unwired: 1 out]
      }
      n2448 = while {
        shift-right: [w7127] -> _
        shift-left: cluster{"Data":string[], "State":T1} {"Data"=[], "State"=enum."PLC通讯初始化"} ("元素") -> [w7128]
        shift-right: [w7134] -> _
        shift-left: w108 -> [w7131]
        shift-right: [w7135] -> _
        shift-left: _ -> [w7132]
        tunnel: w147 -> [w7120]
        tunnel: w145 -> [w7124]
        tunnel: w146 -> [_]
        shift-right: [w7122] -> _
        shift-left: _ -> [w7123]
        stop <- w7125 stop-if-true
        # "OP10"
        n2449 = local read "退出"() -> (w7130:bool)
        n2450 = Wait (ms)(milliseconds to wait=u32 20 ("等待时间（毫秒）")) -> ()  [unwired: 1 out]
        n2451 = Preview Queue Element(queue=w7120) -> (element=→"元素":cluster{"Data":string[], "State":T1})  [unwired: 2 in, 3 out]
        n2452 = call "状态判断.vi"("error IO"=w7131, "退出？"=w7130, "簇 输入"=w7128, "队列输入"=w7120) -> ("error out"=w7118:errorcluster, "簇"=w7129:cluster{"Data":string[], "State":T1})  [unwired: 6 in]
        n2453 = Unbundle By Name(w7129) -> ("Data"=w7126:string[], "State"=w7121:T1)
        "State 10" <- w7121
        n2454 = property on="State 10" class="Enum (严格)"("Val(Sgnl)"=w7121) -> ()  [unwired: 2 in, 2 out]
        n2455 = case shown="\"读数据\"" w7121 {
          tunnel: [w7154 w7185 w7206 w7237 w7258 w7310 w7330 w7412 w7428 w7443 w7463 w7508 w7528 w7582 w7588 w7633 w7661 w7677 refnum<k5> refnum ("TCP") refnum<k5> refnum ("TCP") w7698] -> w7135
          tunnel: [w7136 errorcluster {"status"=FALSE, "code"=0, "source"=""} ("error out") w7186 w7233 w7252 errorcluster {"status"=FALSE, "code"=0, "source"=""} ("error out") w7329 w7392 w7422 errorcluster {"status"=FALSE, "code"=0, "source"=""} ("error out") w7464 w7507 w7524 errorcluster {"status"=FALSE, "code"=0, "source"=""} ("error out") w7587 w7628 w7657 errorcluster {"status"=FALSE, "code"=0, "source"=""} ("error out") errorcluster {"status"=FALSE, "code"=0, "source"=""} ("error out") w7690 w7696] -> w7134
          tunnel: w7132 -> [_ w7185 w7207 w7238 w7259 w7310 w7331 w7380 w7431 w7443 w7447 w7510 w7532 w7582 w7590 w7629 w7665 w7677 w7684 w7691 w7734]
          tunnel: w7120 -> [w7180 _ w7189 _ _ _ w7311 _ _ _ w7461 _ _ _ w7586 _ _ _ w7680 w7692 _]
          tunnel: [cluster{"Data":string[], "State":T1} {"Data"=[], "State"=enum."读扫码请求"} ("元素") cluster{"Data":string[], "State":T1} {"Data"=[], "State"=enum."读扫码请求"} ("元素") w7196 cluster{"Data":string[], "State":T1} {"Data"=[], "State"=enum."读数据保存请求"} ("元素") cluster{"Data":string[], "State":T1} {"Data"=[], "State"=enum."读数据保存请求"} ("元素") cluster{"Data":string[], "State":T1} {"Data"=[], "State"=enum."读数据保存请求"} ("元素") w7319 cluster{"Data":string[], "State":T1} {"Data"=[], "State"=enum."读扫码请求2"} ("元素") cluster{"Data":string[], "State":T1} {"Data"=[], "State"=enum."读扫码请求2"} ("元素") cluster{"Data":string[], "State":T1} {"Data"=[], "State"=enum."读扫码请求2"} ("元素") w7462 cluster{"Data":string[], "State":T1} {"Data"=[], "State"=enum."读数据保存请求2"} ("元素") cluster{"Data":string[], "State":T1} {"Data"=[], "State"=enum."读数据保存请求2"} ("元素") cluster{"Data":string[], "State":T1} {"Data"=[], "State"=enum."读数据保存请求2"} ("元素") w7584 cluster{"Data":string[], "State":T1} {"Data"=[], "State"=enum."看门狗"} ("元素") cluster{"Data":string[], "State":T1} {"Data"=[], "State"=enum."看门狗"} ("元素") cluster{"Data":string[], "State":T1} {"Data"=[], "State"=enum."看门狗"} ("元素") cluster{"Data":string[], "State":T1} {"Data"=[], "State"=enum."PLC通讯初始化"} ("元素") cluster{"Data":string[], "State":T1} {"Data"=[], "State"=enum."退出"} ("元素") cluster{"Data":string[], "State":T1} {"Data"=[], "State"=enum."读扫码请求"} ("元素")] -> w7127
          tunnel: w7126 -> [_ _ _ _ w7257 _ _ _ w7430 _ _ _ w7531 _ _ _ w7663 _ _ _ _]
          tunnel: [FALSE FALSE FALSE FALSE FALSE FALSE FALSE FALSE FALSE FALSE FALSE FALSE FALSE FALSE FALSE FALSE FALSE FALSE FALSE TRUE FALSE] -> w7125
          tunnel: w7124 -> [_ _ _ _ _ _ _ w7404 _ _ _ _ _ _ _ _ _ _ w7681 w7693 _]
          tunnel: w7123 -> [_ w7182 w7190 w7234 w7255 w7306 w7312 w7393 w7425 w7439 w7449 w7509 w7533 w7583 w7589 w7631 w7664 w7678 w7679 w7688 w7727]
          tunnel: [T8 {"扫码2超时"="999", "扫码1超时"="999", "数据保存1超时"="999", "看门狗"="0", "数据保存2超时"="999"} w7182 w7190 w7234 w7254 w7306 w7312 w7393 w7423 w7439 w7448 w7509 w7526 w7583 w7589 w7631 w7659 w7678 w7679 w7688 w7726] -> w7122
          tunnel: w7118 -> [w7137 _ w7187 _ _ _ _ _ _ _ _ _ _ _ _ _ _ _ _ _ _]
          frame "PLC通讯初始化", Default {
            w7141 = u8 0 items=["S7-1200.200.200SMART"=0, "S7-300"=2, "S7-400"=3] ("PLC 系列")
            w7164 = u16 0 items=["byte", "word", "Dword"] ("数据类型")
            w7168 = u8 132 items=["I/O (P)"=128, "Input (I)"=129, "Output (Q)"=130, "Bit Memory (M)"=131, "Data (DB)"=132, "Instance Data (DI)"=133, "Local Data (L)"=134, "Predecessor Local Data (VL)"=135] ("寄存器类型")
            w7159 = u16 0 items=["byte", "word", "Dword"] ("数据类型")
            w7155 = u8 132 items=["I/O (P)"=128, "Input (I)"=129, "Output (Q)"=130, "Bit Memory (M)"=131, "Data (DB)"=132, "Instance Data (DI)"=133, "Local Data (L)"=134, "Predecessor Local Data (VL)"=135] ("寄存器类型")
            # "只需打开一次连接，长连接保持，缩短连接所花时间\n只需要在发生错误的时候再次初始化即可。"
            # "> 增加了时间判定函数，用来记录TCP通讯所用时间 >"
            # "> 所有关于TCP通讯的都需要打时间戳来判定运行时间，也可以用内存运行分析工具来判定。 >"
            n2456 = Enqueue Element(queue=w7180, element=cluster{"Data":string[], "State":T1} {"Data"=["999"], "State"=enum."扫码回复"} ("元素")) -> (queue out=w7176:refnum<queue>, error out=w7175:errorcluster)  [unwired: 2 in, 1 out]
            n2457 = call "S7_Open.vi"("IP 地址"="192.168.0.10", "PLC 系列"=w7141, "超时（MS）"=100, "error in"=w7137) -> ("TCP"=w7139:refnum<k5>, "error out"=w7138:errorcluster)  [unwired: 9 in, 1 out]
            n2458 = Enqueue Element(queue=w7176, element=cluster{"Data":string[], "State":T1} {"Data"=["999"], "State"=enum."扫码回复2"} ("元素"), error in (no error)=w7175) -> (queue out=w7174:refnum<queue>, error out=w7173:errorcluster)  [unwired: 1 in, 1 out]
            n2459 = Unbundle By Name(w7138) -> ("status"=→"ST10通讯状态":bool)
            n2460 = call "S7_Read.vi"("TCP"=w7139, "DB #"=u16 20, "读取长度"=u16 17, "寄存器类型"=w7155, "起始地址"=u32 24, "数据类型"=w7159, "error in"=w7138) -> ("TCP"=w7169:refnum<k5>, "数据"=w7160:u32[], "error out"=w7144:errorcluster)  [unwired: 5 in, 1 out]
            n2461 = Enqueue Element(queue=w7174, element=cluster{"Data":string[], "State":T1} {"Data"=["999"], "State"=enum."数据保存回复"} ("元素"), error in (no error)=w7173) -> (queue out=w7152:refnum<queue>, error out=w7151:errorcluster)  [unwired: 1 in, 1 out]
            n2462 = To Unsigned Word Integer(number=w7160) -> (unsigned 16bit integer=w7161:u16[])
            n2463 = call "还原为字符串.vi"("输入数组"=w7161) -> ("字符串"=w7149:string)  [unwired: 9 in, 1 out]
            n2464 = Match Pattern(string=w7149, regular expression=" " ("正则表达式")) -> (before substring=w7148:string)  [unwired: 1 in, 3 out]
            n2465 = local write "101 二维码"(w7148) -> ()
            n2466 = Enqueue Element(queue=w7152, element=cluster{"Data":string[], "State":T1} {"Data"=["999"], "State"=enum."数据保存回复2"} ("元素"), error in (no error)=w7151) -> ()  [unwired: 1 in, 3 out]
            n2467 = call "S7_Read.vi"("TCP"=w7169, "DB #"=u16 20, "读取长度"=u16 17, "寄存器类型"=w7168, "起始地址"=u32 42, "数据类型"=w7164, "error in"=w7144) -> ("TCP"=w7154:refnum<k5>, "数据"=w7163:u32[], "error out"=w7136:errorcluster)  [unwired: 5 in, 1 out]
            n2468 = To Unsigned Word Integer(number=w7163) -> (unsigned 16bit integer=w7162:u16[])
            n2469 = call "还原为字符串.vi"("输入数组"=w7162) -> ("字符串"=w7146:string)  [unwired: 9 in, 1 out]
            n2470 = Match Pattern(string=w7146, regular expression=" " ("正则表达式")) -> (before substring=w7145:string)  [unwired: 1 in, 3 out]
            n2471 = local write "102 二维码"(w7145) -> ()
          }
          frame "---------------" {
          }
          frame "读扫码请求" {
            w7215 = u16 0 items=["byte", "word", "Dword"] ("数据类型")
            w7217 = u8 132 items=["I/O (P)"=128, "Input (I)"=129, "Output (Q)"=130, "Bit Memory (M)"=131, "Data (DB)"=132, "Instance Data (DI)"=133, "Local Data (L)"=134, "Predecessor Local Data (VL)"=135] ("寄存器类型")
            n2472 = call "S7_Read.vi"("TCP"=w7207, "DB #"=u16 20, "读取长度"=u16 1, "寄存器类型"=w7217, "起始地址"=u32 0, "数据类型"=w7215, "error in"=w7187) -> ("TCP"=w7206:refnum<k5>, "数据"=w7212:u32[], "error out"=w7186:errorcluster)  [unwired: 5 in, 1 out]
            n2473 = Index Array(array=w7212, index=0 ("索引")) -> (element=w7210:u32)
            n2474 = Number To Boolean Array(number=w7210) -> (Boolean array=w7209:bool[])
            n2475 = Index Array(array=w7209, index=0 ("索引")) -> (element=w7188:bool)
            "ST101扫码请求" <- w7188
            n2476 = Unbundle By Name(w7190) -> ("扫码1超时"=w7191:string)
            n2477 = Not Equal?(x=w7191, y="999") -> (x != y?=w7193:bool)
            n2478 = Not(x=w7193) -> (.not. x?=w7194:bool)
            n2479 = call <vilib>:"Boolean Crossing PtByPt.vi"("direction"=enum16{"either", "false-true", "true-false"}."false-true", "input"=w7188) -> ("crossing"=w7202:bool)  [unwired: 1 in]
            n2480 = call <vilib>:"Boolean Crossing PtByPt.vi"("direction"=enum16{"either", "false-true", "true-false"}."true-false", "input"=w7188) -> ("crossing"=w7201:bool)  [unwired: 1 in]
            n2481 = call "已用时间3"("Reset"=w7194) -> ("Time has Elapsed"=w7195:bool)  [unwired: 11 in, 7 out]
            n2482 = Insert Into Array(array=bool[] [] ("数组"), index=0 ("索引"), new element #1=w7202, new element #2=w7201) -> (w7198:bool[])
            n2483 = Boolean Array To Number(Boolean array=w7198) -> (number=w7197:u32)
            n2484 = case shown="0, 默认" w7197 {
              tunnel: [cluster{"Data":string[], "State":T1} {"Data"=[], "State"=enum."读数据保存请求"} ("元素") w7223 w7226] -> w7196
              tunnel: w7189 -> [_ w7224 w7227]
              frame 0, Default {
              }
              frame 1 {
                w7223 = cluster{"Data":string[], "State":T1} {"Data"=[], "State"=enum."读二维码"} ("元素")
                n2485 = Enqueue Element(queue=w7224, element=w7223, timeout in ms (-1)=10 ("超时毫秒(-1)")) -> ()  [unwired: 1 in, 3 out]
              }
              frame 2 {
                w7226 = cluster{"Data":string[], "State":T1} {"Data"=["999"], "State"=enum."扫码回复"} ("元素")
                n2486 = Enqueue Element(queue=w7227, element=w7226, timeout in ms (-1)=10 ("超时毫秒(-1)")) -> ()  [unwired: 1 in, 3 out]
              }
            }
            n2487 = case shown="真" w7195 {
              tunnel: w7189 -> [_ w7219]
              frame False {
              }
              frame True {
                n2488 = Enqueue Element(queue=w7219, element=cluster{"Data":string[], "State":T1} {"Data"=["999"], "State"=enum."扫码回复"} ("元素"), timeout in ms (-1)=10 ("超时毫秒(-1)")) -> ()  [unwired: 1 in, 3 out]
              }
            }
          }
          frame "读二维码" {
            w7243 = u16 0 items=["byte", "word", "Dword"] ("数据类型")
            w7239 = u8 132 items=["I/O (P)"=128, "Input (I)"=129, "Output (Q)"=130, "Bit Memory (M)"=131, "Data (DB)"=132, "Instance Data (DI)"=133, "Local Data (L)"=134, "Predecessor Local Data (VL)"=135] ("寄存器类型")
            n2489 = call "S7_Read.vi"("TCP"=w7238, "DB #"=u16 20, "读取长度"=u16 17, "寄存器类型"=w7239, "起始地址"=u32 24, "数据类型"=w7243) -> ("TCP"=w7237:refnum<k5>, "数据"=w7244:u32[], "error out"=w7246:errorcluster)  [unwired: 6 in, 1 out]
            n2490 = To Unsigned Word Integer(number=w7244) -> (unsigned 16bit integer=w7245:u16[])
            n2491 = call "还原为字符串.vi"("error in (no error)"=w7246, "输入数组"=w7245) -> ("error out"=w7230:errorcluster, "字符串"=w7231:string)  [unwired: 8 in]
            n2492 = Match Pattern(string=w7231, regular expression=" " ("正则表达式")) -> (before substring=w7228:string)  [unwired: 1 in, 3 out]
            n2493 = flat-sequence {
              tunnel: w7230 -> [w7248]
              tunnel: [w7248] -> w7229
              tunnel: w7228 -> [w7247]
              tunnel: [w7250] -> w7233
              tunnel: w7229 -> [w7249]
              frame #0 {
                "101 二维码" <- w7247
              }
              frame #1 {
                n2494 = property on="ST101扫码请求（事件）" class="Bool (严格)"(error in=w7249, "Val(Sgnl)"=TRUE ("值(信号)")) -> (error out=w7250:errorcluster)  [unwired: 1 in, 1 out]
              }
            }
          }
          frame "扫码回复" {
            n2495 = Array Size(array=w7257) -> (size(s)=w7256:i32)
            n2496 = case shown="3, 默认" w7256 {
              tunnel: w7259 -> [w7274 w7297]
              tunnel: [w7265 w7299] -> w7258
              tunnel: [w7264 w7298] -> w7252
              tunnel: w7257 -> [w7263 w7296]
              tunnel: [w7262 w7294] -> w7253
              frame 3, Default {
                w7277 = u8 132 items=["I/O (P)"=128, "Input (I)"=129, "Output (Q)"=130, "Bit Memory (M)"=131, "Data (DB)"=132, "Instance Data (DI)"=133, "Local Data (L)"=134, "Predecessor Local Data (VL)"=135] ("寄存器类型")
                w7276 = u16 1 items=["byte", "word", "Dword"] ("数据类型")
                w7284 = u8 132 items=["I/O (P)"=128, "Input (I)"=129, "Output (Q)"=130, "Bit Memory (M)"=131, "Data (DB)"=132, "Instance Data (DI)"=133, "Local Data (L)"=134, "Predecessor Local Data (VL)"=135] ("寄存器类型")
                w7285 = u16 1 items=["byte", "word", "Dword"] ("数据类型")
                w7290 = u8 132 items=["I/O (P)"=128, "Input (I)"=129, "Output (Q)"=130, "Bit Memory (M)"=131, "Data (DB)"=132, "Instance Data (DI)"=133, "Local Data (L)"=134, "Predecessor Local Data (VL)"=135] ("寄存器类型")
                w7289 = u16 1 items=["byte", "word", "Dword"] ("数据类型")
                n2497 = Index Array(array=w7263) -> (element #1=w7262:string, element #2=w7270:string, element #3=w7269:string)  [unwired: 3 in]
                n2498 = Equal?(x=w7269, y="OK") -> (x = y?=w7267:bool)
                n2499 = Decimal String To Number(string=w7270, default (0L)=u32 0 ("默认(0 I32)")) -> (number=w7271:u32)  [unwired: 1 in, 1 out]
                n2500 = case shown="真" w7267 {
                  tunnel: [u32 2 ("写入数据") u32 1 ("写入数据")] -> w7266
                  frame False {
                  }
                  frame True {
                  }
                }
                n2501 = call "S7_Write.vi"("TCP"=w7274, "寄存器类型"=w7290, "DB #"=u16 20, "写入地址"=u32 8, "数据类型"=w7289, "写入数据"=w7271) -> ("TCP"=w7281:refnum<k5>, "error out"=w7282:errorcluster)  [unwired: 7 in, 1 out]
                n2502 = call "S7_Write.vi"("TCP"=w7281, "寄存器类型"=w7284, "DB #"=u16 20, "写入地址"=u32 10, "数据类型"=w7285, "写入数据"=w7266, "error in"=w7282) -> ("TCP"=w7273:refnum<k5>, "error out"=w7272:errorcluster)  [unwired: 6 in, 1 out]
                n2503 = Decimal String To Number(string=w7262, default (0L)=u32 0 ("默认(0 I32)")) -> (number=w7280:u32)  [unwired: 1 in, 1 out]
                n2504 = call "S7_Write.vi"("TCP"=w7273, "寄存器类型"=w7277, "DB #"=u16 20, "写入地址"=u32 2, "数据类型"=w7276, "写入数据"=w7280, "error in"=w7272) -> ("TCP"=w7265:refnum<k5>, "error out"=w7264:errorcluster)  [unwired: 6 in, 1 out]
              }
              frame 1 {
                w7302 = u8 132 items=["I/O (P)"=128, "Input (I)"=129, "Output (Q)"=130, "Bit Memory (M)"=131, "Data (DB)"=132, "Instance Data (DI)"=133, "Local Data (L)"=134, "Predecessor Local Data (VL)"=135] ("寄存器类型")
                w7301 = u16 1 items=["byte", "word", "Dword"] ("数据类型")
                n2505 = Index Array(array=w7296, index=0 ("索引")) -> (element=w7294:string)
                n2506 = Decimal String To Number(string=w7294, default (0L)=u32 0 ("默认(0 I32)")) -> (number=w7305:u32)  [unwired: 1 in, 1 out]
                n2507 = call "S7_Write.vi"("TCP"=w7297, "寄存器类型"=w7302, "DB #"=u16 20, "写入地址"=u32 2, "数据类型"=w7301, "写入数据"=w7305) -> ("TCP"=w7299:refnum<k5>, "error out"=w7298:errorcluster)  [unwired: 7 in, 1 out]
              }
            }
            "扫码请求回复101" <- w7253
            n2508 = Bundle By Name(cluster=w7255, "扫码1超时"=w7253) -> (w7254:T8)
          }
          frame "-------------" {
          }
          frame "读数据保存请求" {
            w7339 = u16 0 items=["byte", "word", "Dword"] ("数据类型")
            w7341 = u8 132 items=["I/O (P)"=128, "Input (I)"=129, "Output (Q)"=130, "Bit Memory (M)"=131, "Data (DB)"=132, "Instance Data (DI)"=133, "Local Data (L)"=134, "Predecessor Local Data (VL)"=135] ("寄存器类型")
            n2509 = call "S7_Read.vi"("TCP"=w7331, "DB #"=u16 20, "读取长度"=u16 1, "寄存器类型"=w7341, "起始地址"=u32 0, "数据类型"=w7339) -> ("TCP"=w7330:refnum<k5>, "数据"=w7336:u32[], "error out"=w7329:errorcluster)  [unwired: 6 in, 1 out]
            n2510 = Index Array(array=w7336, index=0 ("索引")) -> (element=w7334:u32)
            n2511 = Number To Boolean Array(number=w7334) -> (Boolean array=w7333:bool[])
            n2512 = Unbundle By Name(w7312) -> ("数据保存1超时"=w7313:string)
            n2513 = Index Array(array=w7333, index=1 ("索引")) -> (element=w7318:bool)
            "ST101数据读取" <- w7318
            n2514 = Not Equal?(x=w7313, y="999") -> (x != y?=w7315:bool)
            n2515 = Not(x=w7315) -> (.not. x?=w7316:bool)
            n2516 = call <vilib>:"Boolean Crossing PtByPt.vi"("direction"=enum16{"either", "false-true", "true-false"}."false-true", "input"=w7318) -> ("crossing"=w7322:bool)  [unwired: 1 in]
            n2517 = call <vilib>:"Boolean Crossing PtByPt.vi"("direction"=enum16{"either", "false-true", "true-false"}."true-false", "input"=w7318) -> ("crossing"=w7323:bool)  [unwired: 1 in]
            n2518 = call "已用时间4"("Reset"=w7316) -> ("Time has Elapsed"=w7317:bool)  [unwired: 11 in, 7 out]
            n2519 = Insert Into Array(array=bool[] [] ("数组"), index=0 ("索引"), new element #1=w7322, new element #2=w7323) -> (w7326:bool[])
            n2520 = Boolean Array To Number(Boolean array=w7326) -> (number=w7327:u32)
            n2521 = case shown="2" w7327 {
              tunnel: [cluster{"Data":string[], "State":T1} {"Data"=[], "State"=enum."读扫码请求2"} ("元素") w7347 w7349] -> w7319
              tunnel: w7311 -> [_ w7348 w7350]
              frame 0, Default {
              }
              frame 1 {
                w7347 = cluster{"Data":string[], "State":T1} {"Data"=[], "State"=enum."读数据"} ("元素")
                n2522 = Enqueue Element(queue=w7348, element=w7347, timeout in ms (-1)=10 ("超时毫秒(-1)")) -> ()  [unwired: 1 in, 3 out]
              }
              frame 2 {
                w7349 = cluster{"Data":string[], "State":T1} {"Data"=["999"], "State"=enum."数据保存回复"} ("元素")
                n2523 = Enqueue Element(queue=w7350, element=w7349, timeout in ms (-1)=10 ("超时毫秒(-1)")) -> ()  [unwired: 1 in, 3 out]
              }
            }
            n2524 = case shown="真" w7317 {
              tunnel: w7311 -> [_ w7343]
              frame False {
              }
              frame True {
                n2525 = Enqueue Element(queue=w7343, element=cluster{"Data":string[], "State":T1} {"Data"=["999"], "State"=enum."数据保存回复"} ("元素"), timeout in ms (-1)=10 ("超时毫秒(-1)")) -> ()  [unwired: 1 in, 3 out]
              }
            }
          }
          frame "读数据" {
            w7370 = u16 2 items=["byte", "word", "Dword"] ("数据类型")
            w7366 = u8 132 items=["I/O (P)"=128, "Input (I)"=129, "Output (Q)"=130, "Bit Memory (M)"=131, "Data (DB)"=132, "Instance Data (DI)"=133, "Local Data (L)"=134, "Predecessor Local Data (VL)"=135] ("寄存器类型")
            w7385 = u16 0 items=["byte", "word", "Dword"] ("数据类型")
            w7381 = u8 132 items=["I/O (P)"=128, "Input (I)"=129, "Output (Q)"=130, "Bit Memory (M)"=131, "Data (DB)"=132, "Instance Data (DI)"=133, "Local Data (L)"=134, "Predecessor Local Data (VL)"=135] ("寄存器类型")
            w7413 = u16 1 items=["byte", "word", "Dword"] ("数据类型")
            w7417 = u8 132 items=["I/O (P)"=128, "Input (I)"=129, "Output (Q)"=130, "Bit Memory (M)"=131, "Data (DB)"=132, "Instance Data (DI)"=133, "Local Data (L)"=134, "Predecessor Local Data (VL)"=135] ("寄存器类型")
            n2526 = call "S7_Read.vi"("TCP"=w7380, "DB #"=u16 20, "读取长度"=u16 1, "寄存器类型"=w7381, "起始地址"=u32 0, "数据类型"=w7385) -> ("TCP"=w7365:refnum<k5>, "数据"=w7375:u32[], "error out"=w7364:errorcluster)  [unwired: 6 in, 1 out]
            n2527 = Index Array(array=w7375, index=0 ("索引")) -> (element=w7379:u32)
            n2528 = Number To Boolean Array(number=w7379) -> (Boolean array=w7378:bool[])
            n2529 = Index Array(array=w7378, index=4 ("索引")) -> (element=w7374:bool)
            n2530 = call "S7_Read.vi"("TCP"=w7365, "DB #"=u16 20, "读取长度"=u16 4, "寄存器类型"=w7366, "起始地址"=u32 220, "数据类型"=w7370, "error in"=w7364) -> ("TCP"=w7363:refnum<k5>, "数据"=w7360:u32[], "error out"=w7362:errorcluster)  [unwired: 5 in, 1 out]
            n2531 = Equal?(x=w7374, y=TRUE) -> (x = y?=w7372:bool)
            n2532 = Index Array(array=w7360, index #1=0 ("索引")) -> (element #1=w7356:u32, element #2=w7359:u32, element #3=w7358:u32, element #4=w7357:u32)  [unwired: 3 in]
            n2533 = case shown="真" w7372 {
              tunnel: [" " "Y"] -> w7371
              frame False {
              }
              frame True {
              }
            }
            n2534 = Number To Decimal String(number=w7356) -> (decimal integer string=w7355:string)  [unwired: 1 in]
            n2535 = Number To Decimal String(number=w7359) -> (decimal integer string=w7353:string)  [unwired: 1 in]
            n2536 = Number To Decimal String(number=w7358) -> (decimal integer string=w7354:string)  [unwired: 1 in]
            n2537 = Number To Decimal String(number=w7357) -> (decimal integer string=w7352:string)  [unwired: 1 in]
